vi "PH_Sixpack.ProcCases.vi"(0 "i ref in":refnum<vi>, 1 "selector":string, 2 "Data":T1, 3 "call cluster":T2={"Object"="", "Selector"="", "CallType"=enum."synchronous", "Async Object"="", "Async Selector"="", "Data Descriptor"="", "Data"=[], "Error #"=0, "Expire"=0}, 5 "error in":errorcluster) -> (14 "i ref out":refnum<vi>, 17 "answer cluster":T2={"Object"="", "Selector"="", "CallType"=enum."synchronous", "Async Object"="", "Async Selector"="", "Data Descriptor"="", "Data"=[], "Error #"=0, "Expire"=0}, 19 "error out":errorcluster)   [LabVIEW 2014, in "PH_Sixpack.lvlib"]
doc: "This method is called by a process from within the default case in the event loop. The methods of a class that are linked to events will be called from THIS method. Add your code here."
uses:
  PH_Sixpack.lvlib
  CSCore/CSSystem/CoreDefs/CoreDefs.call_type.ctl
  CSCore/BaseProcess/BaseProcess.descriptor string definition.ctl
  CSCore/CSSystem/CoreDefs/CoreDefs.rawDataType.ctl
  PH_Sixpack.Status.ctl
  PH_PSDBWriter/PH_PSDBWriter.Thread Commands.ctl
  instr.lib/SixPack/PackDLL/Current Control.ctl
  instr.lib/SixPack/PackDLL/Current.ctl
  instr.lib/SixPack/PackDLL/VStartVmin.ctl
  instr.lib/SixPack/PackDLL/VmaxAmax.ctl
  instr.lib/SixPack/PackDLL/MotorParameter_P5.ctl
  instr.lib/SixPack/PackDLL/MotorParameter_P6.ctl
  instr.lib/SixPack/PackDLL/Motor Parameter.ctl
  instr.lib/SixPack/PackDLL/Ref Search Parameter.ctl
  instr.lib/SixPack/PackDLL/Stopswitch Limits.ctl
  CSCore/CSSystem/CoreLib/CoreLib.string 2 byte array.vi
  CSCore/CSSystem/CoreLib/CoreLib.byte array 2 int.vi
  CSCore/CSSystem/CoreLib/CoreLib.byte array 2 double.vi
  CSCore/CSSystem/CoreLib/CoreLib.lvlib
  CSCore/BaseProcess/BaseProcess.lvlib
  CSCore/CAEObj/CAEObj.lvlib
  PH_PSDBWriter/PH_PSDBWriter.lvlib
  PH_Stepmotor_BaseClass/PH_Stepmotor_BaseClass.lvlib
  instr.lib/SixPack/Sixpack - Driver.lvlib
  CSCore/CSSystem/CSSystemLib/CSSystemLib.lvlib
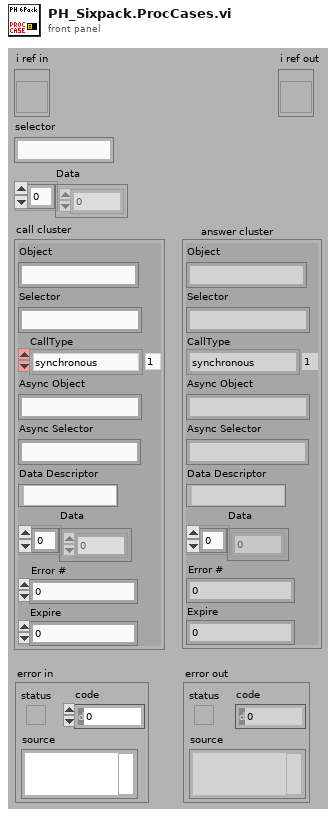
[diagram p1: front panel]
types:
  T1 = typedef "CoreDefs.rawDataType.ctl" = i8[]
  T2 = typedef "CoreDefs.call_type.ctl" = cluster{"Object":string, "Selector":string, "CallType":enum16{"simple", "synchronous", "asynchronous"}, "Async Object":string, "Async Selector":string, "Data Descriptor":T3, "Data":T1, "Error #":i32, "Expire":u32}
  T3 = typedef "BaseProcess.lvlib/BaseProcess.descriptor string definition.ctl" = string
  T4 = typedef "PH_Sixpack.lvlib/PH_Sixpack.Status.ctl" = enum32{"None", "Init", "Configure", "configured", "Close", "closed"}
  T5 = typedef "Sixpack - Driver.lvlib/Current Control.ctl" = cluster{"PowerDownDelay (500)":u16, "PowerDown (0%)":T6, "Standing (50%)":T6, "Running (75%)":T6, "Accelerating (100%)":T6}
  T6 = typedef "Sixpack - Driver.lvlib/Current.ctl" = enum8{"100%", "75%", "50%", "38%", "25%", "19%", "13%", "9%", "0%"}
  T7 = typedef "Sixpack - Driver.lvlib/VStartVmin.ctl" = cluster{"VStart(5)":u16, "Vmin(4)":u16, "Div i (2)":enum8{"0", "1", "2", "3"}}
  T8 = typedef "Sixpack - Driver.lvlib/VmaxAmax.ctl" = cluster{"VMax(511)":u16, "AMax(128)":u16}
  T9 = typedef "Sixpack - Driver.lvlib/Motor Parameter.ctl" = cluster{"Poslimit (6400)":u32, "P5 Bits":T10, "P6 Bits":T11}
  T10 = typedef "Sixpack - Driver.lvlib/MotorParameter_P5.ctl" = cluster{"MT_PI":bool, "MT_ROTARY":bool, "MT_AUTONULLCMD":bool, "MT_TESTNULL":bool, "MT_NULLLEFT":bool, "MT_NULLCENTRE":bool, "MT_STOPNULL":bool, "MT_FILTERSWITCH":bool}
  T11 = typedef "Sixpack - Driver.lvlib/MotorParameter_P6.ctl" = cluster{"MT_OPTIMIZEWAY":bool, "MT_FASTREF":bool, "MT_MECHREF":bool, "MT_DELAYTESTNULL":bool, "MT_STOPSOFT":bool, "MT_STOPNOREF":bool, "MT_NULLPOSITIVE":bool, "MUT_STOPFULSTEPS":bool}
  T12 = typedef "Sixpack - Driver.lvlib/Ref Search Parameter.ctl" = cluster{"VRefMax(100)":u16, "DebouncingTime (22ms)":u8}
  T13 = typedef "Sixpack - Driver.lvlib/Stopswitch Limits.ctl" = cluster{"MinLeft(0)":u16, "MaxRight(1023)":u16}
  T14 = typedef "PH_PSDBWriter.lvlib/PH_PSDBWriter.PHELIX-Subsystems.ctl" = i32
  T15 = typedef "PH_PSDBWriter.lvlib/PH_PSDBWriter.Thread Commands.ctl" = u16
  T16 = typedef "PH_Stepmotor_BaseClass.lvlib/PH_Stepmotor_BaseClass.i attribute.ctl" = cluster{"Device Error":errorcluster, "Axes PSDB Thread":cluster{"Ref":refnum<vi>, "Q-Ref":refnum<queue>, "Data Status":T17}, "Axes":T18[], "Axes PSDB Infos":cluster{"GUI Name":string, "PSDB Instance ID":i32, "PSDB Status Service ID":i32, "Axis":i32, "Class":string}[], "GUI Refs":T23}
  T17 = typedef "PH_PSDBWriter.lvlib/PH_PSDBWriter.Data Status.ctl" = i16
  T18 = typedef "PH_Stepmotor_BaseClass.lvlib/PH_Stepmotor_BaseClass.Axis Attributes.ctl" = cluster{"Settings":T19, "Endswitch?":bool, "DIM Service IDs":T21, "Activity":T22, "Configured?":bool, "Position":cluster{"Current":i32, "Target":i32}, "Position to set":cluster{"New?":bool, "Wanted":i32}, "Stop?":bool, "Reset?":bool, "Move?":bool, "Nothing connected?":bool}
  T19 = typedef "PH_Stepmotor_BaseClass.lvlib/PH_Stepmotor_BaseClass.Axis Settings.ctl" = cluster{"Sign change":bool, "Width":dbl, "Calibration":dbl, "Unit":string, "Motor Type":T20, "Unit Width":string, "Unit CF":string}
  T20 = typedef "PH_Stepmotor_BaseClass.lvlib/PH_Stepmotor_BaseClass.Motor Type.ctl" = enum16{"Unspecific", "OWIS 49.120.2633", "OWIS 49.060.1033", "OWIS 43.040.2558", "Diamond Motion 2200 series", "OWIS 49.120.266B.MV6", "Calorimeter", "Linear Stage 1", "MICOS VT-80", "MICOS VT-80 S", "Standa Rotstage nt0.95A", "PUF RA 320.200", "PUF RA 800.200", "PUF RA 800.400", "PUF RA 400.50", "1324.nn.800.50", "1324.n9c.800.50", "1324.nn.320.200", "1324.nn.400.200", "1324.nn.800.200", "1324.nn.400.50", "1324.8c9c.800.50", "1324.8c9c.400.200"}
  T21 = typedef "PH_Stepmotor_BaseClass.lvlib/PH_Stepmotor_BaseClass.Axis DIM Service IDs.ctl" = cluster{"Settings":i32, "Information":i32}
  T22 = typedef "PH_Stepmotor_BaseClass.lvlib/PH_Stepmotor_BaseClass.Axis Activity.ctl" = enum16{"No Information", "stopped", "running", "Failure", "Alarm", "stopped at backward ES", "stopped at foreward ES"}
  T23 = typedef "PH_Stepmotor_BaseClass.lvlib/PH_Stepmotor_BaseClass.GUI Refs.ctl" = cluster{"Axes Configuration":refnum<vi>, "Device Error":refnum<vi>, "Axes PSDB Infos":refnum<vi>}
  T24 = cluster{"Boolean array[0]":bool, "Boolean array[1]":bool, "Boolean array[2]":bool, "Boolean array[3]":bool, "Boolean array[4]":bool, "Boolean array[5]":bool, "Boolean array[6]":bool, "Boolean array[7]":bool}
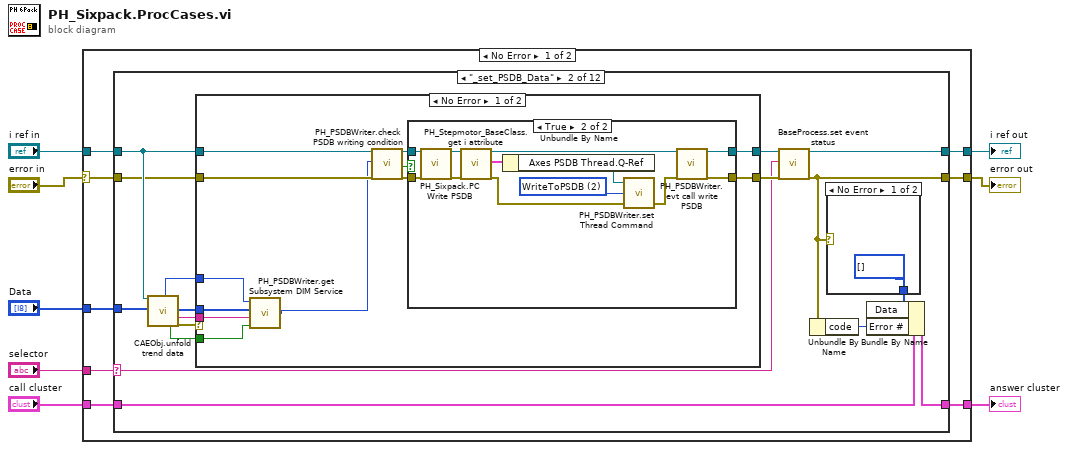
[diagram p0: block diagram]
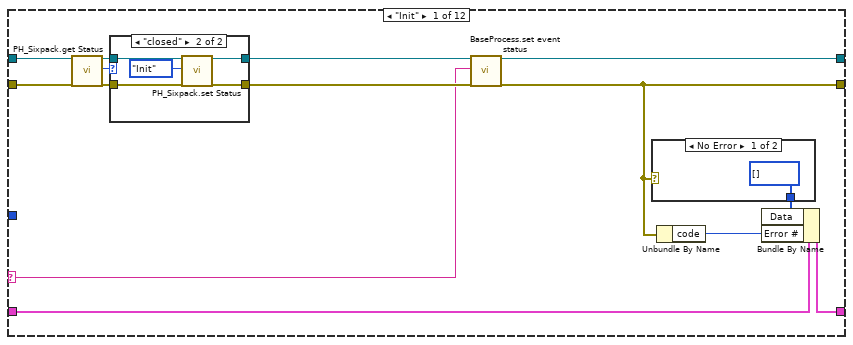
[diagram p2: hidden frame]
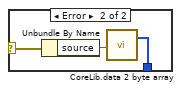
[diagram p4: hidden frame]
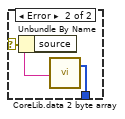
[diagram p7: hidden frame]
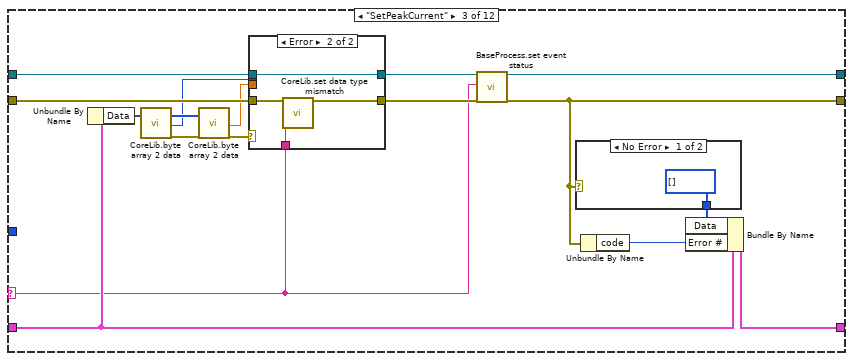
[diagram p8: hidden frame]
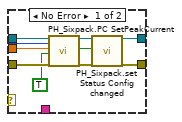
[diagram p9: hidden frame]
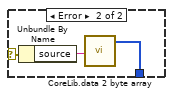
[diagram p10: hidden frame]
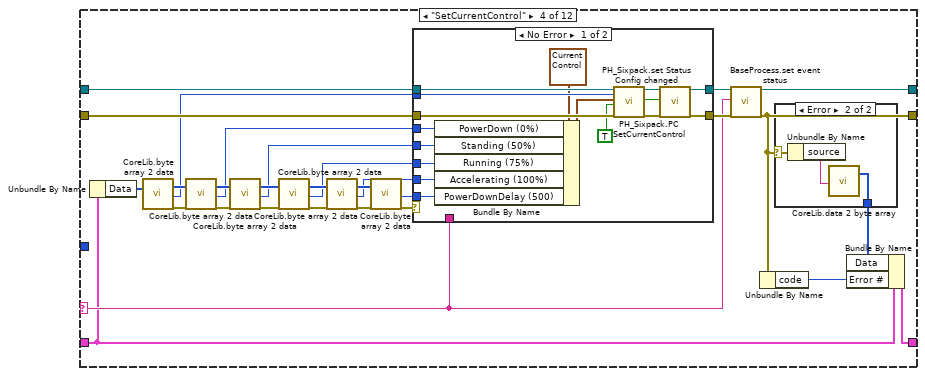
[diagram p11: hidden frame]
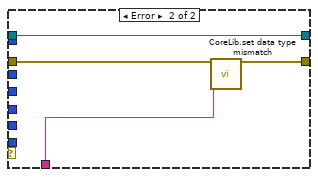
[diagram p12: hidden frame]
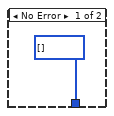
[diagram p13: hidden frame]
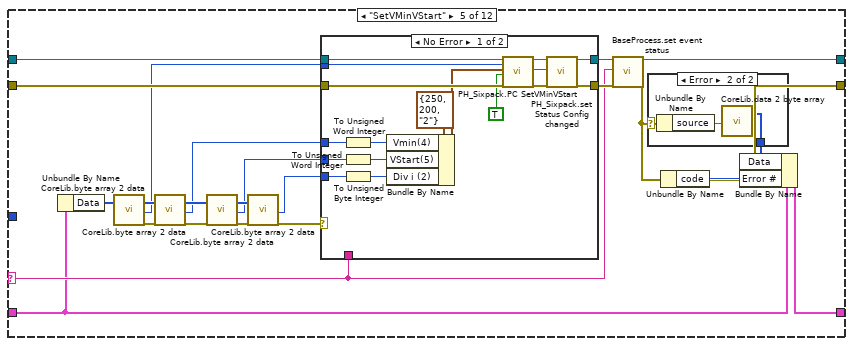
[diagram p14: hidden frame]
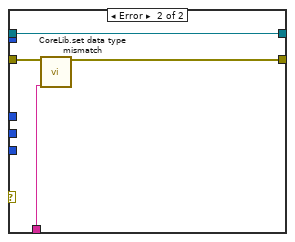
[diagram p15: hidden frame]
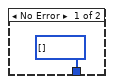
[diagram p16: hidden frame]
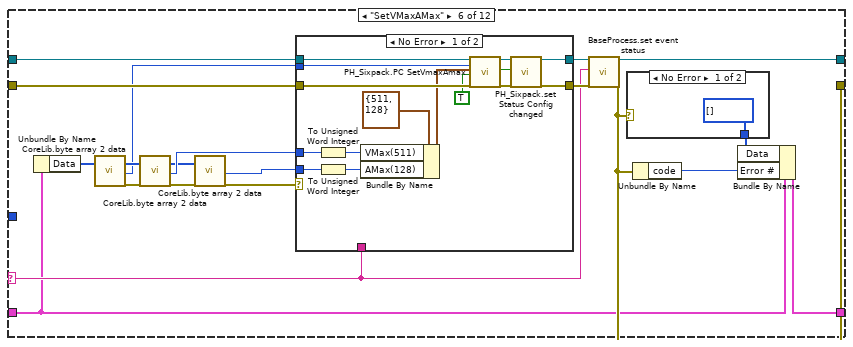
[diagram p17: hidden frame]
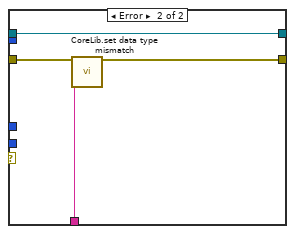
[diagram p18: hidden frame]
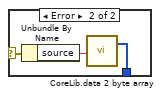
[diagram p19: hidden frame]
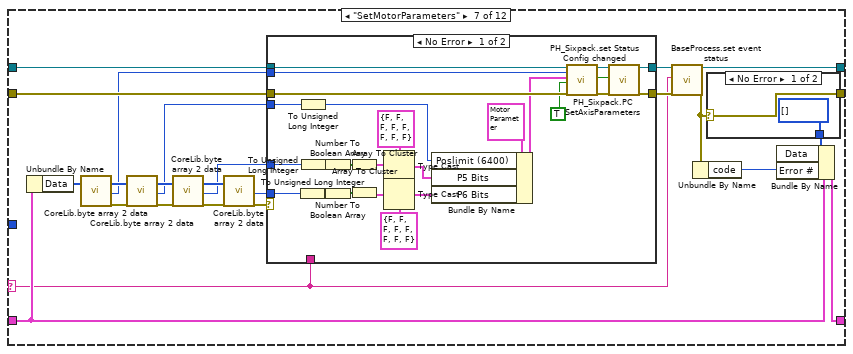
[diagram p20: hidden frame]
diagram:
  n1 = case shown="No Error" "error in" {
    selector: "error in" -> [w11 w500]
    tunnel: [w16 w499] -> w8
    tunnel: [w9 w500] -> w7
    tunnel: "call cluster" -> [w15 w499]
    tunnel: "selector" -> [w14 _]
    tunnel: [w10 w501] -> w4
    tunnel: "i ref in" -> [w13 w501]
    tunnel: "Data" -> [w12 _]
    frame No Error {
      n2 = case shown="\"_set_PSDB_Data\"" w14 {
        selector: w14 -> [w22 w43 w99 w149 w194 w239 w270 w337 w382 w419 w458 w474]
        tunnel: [w25 w56 w104 w151 w198 w242 w289 w342 w385 w422 w459 w484] -> w10
        tunnel: w15 -> [w30 w44 w100 w148 w193 w238 w286 w341 w381 w418 w462 w486]
        tunnel: [w29 w58 w102 w147 w195 w246 w287 w340 w369 w413 w461 w489] -> w16
        tunnel: w11 -> [w27 w47 w103 w150 w197 w244 w288 w339 w384 w421 w455 w490]
        tunnel: [w23 w55 w101 w146 w196 w240 w273 w338 w383 w420 w456 w482] -> w9
        tunnel: w13 -> [w19 w48 w98 w145 w192 w237 w285 w336 w380 w417 w452 w488]
        tunnel: w12 -> [_ w42 _ _ _ _ _ _ _ _ _ w487]
        frame "Init" {
          n3 = call "PH_Sixpack.get Status.vi"("VI in"=w19, "error in (no error)"=w27) -> ("VI out"=w18:refnum<vi>, "Status"=w17:T4, "Device Error"=w20:errorcluster)  [unwired: 14 in, 1 out]
          n4 = case shown="\"closed\"" w17 {
            tunnel: [w32 w37] -> w26
            tunnel: [w31 w36] -> w24
            tunnel: w20 -> [w31 w34]
            tunnel: w18 -> [w32 w33]
            frame "None", Default {
            }
            frame "closed" {
              n5 = call "PH_Sixpack.set Status.vi"("VI in"=w33, "Status"=PH_Sixpack.Status."Init", "error in (no error)"=w34) -> ("VI out"=w37:refnum<vi>, "error out"=w36:errorcluster)  [unwired: 15 in]
            }
          }
          n6 = call "BaseProcess.set event status.vi"("i ref in"=w26, "EventStatus"=w22, "error in (no error)"=w24) -> ("i ref out"=w25:refnum<vi>, "error out"=w23:errorcluster)  [unwired: 14 in, 1 out]
          n7 = case shown="No Error" w23 {
            selector: w23 -> [_ w41]
            tunnel: [T1 [] ("byteArray out") w39] -> w21
            frame No Error {
            }
            frame Error {
              n8 = Unbundle By Name(w41) -> ("source"=w40:string)
              n9 = call-poly "CoreLib.data 2 byte array.vi"("string"=w40) -> ("byteArray out"=w39:T1)  [unwired: 18 in]
            }
          }
          n10 = Unbundle By Name(w23) -> ("code"=w28:i32)
          n11 = Bundle By Name(cluster=w30, "Data"=w21, "Error #"=w28) -> (w29:T2)
        }
        frame "_set_PSDB_Data" {
          n12 = call "CAEObj.unfold trend data.vi"("i ref in"=w48, "raw trend data"=w42) -> ("quality"=w49:i32, "no link"=w52:bool, "data"=w50:i8[], "typeDescriptor"=w51:string, "error out"=w53:errorcluster)  [unwired: 9 in, 4 out]
          n13 = case shown="No Error" w53 {
            tunnel: w47 -> [w70 w86]
            tunnel: [w69 w85] -> w46
            tunnel: [w68 w86] -> w45
            tunnel: w48 -> [w66 w85]
            tunnel: w52 -> [w60 _]
            tunnel: w51 -> [w61 _]
            tunnel: w50 -> [w63 _]
            tunnel: w49 -> [w62 _]
            frame No Error {
              n14 = call "PH_PSDBWriter.get Subsystem DIM Service.vi"("no link"=w60, "typeDescriptor"=w61, "data"=w63, "quality"=w62) -> ("PHELIX Subsystems"=w59:T14)
              n15 = call "PH_PSDBWriter.check PSDB writing condition.vi"("i ref in"=w66, "wanted Subsystem"=w59, "error IO"=w70) -> ("i ref out"=w65:refnum<vi>, "write PSDB?"=w64:bool, "error out"=w67:errorcluster)  [unwired: 14 in]
              n16 = case shown="True" w64 {
                tunnel: w67 -> [w71 w84]
                tunnel: [w72 w75] -> w69
                tunnel: [w71 w73] -> w68
                tunnel: w65 -> [w72 w83]
                frame False {
                }
                frame True {
                  w79 = T15 2 items=["None", "GetInstanceID", "WriteToPSDB"] ("PSDB Thread Command")
                  n17 = call "PH_Sixpack.PC Write PSDB.vi"("i ref in"=w83, "error IO"=w84) -> ("i ref out"=w77:refnum<vi>, "error out"=w78:errorcluster)  [unwired: 16 in]
                  n18 = call "PH_Stepmotor_BaseClass.get i attribute.vi"("i ref in"=w77, "error in (no error)"=w78) -> ("i ref out"=w76:refnum<vi>, "i attribute"=w81:T16, "error out"=w82:errorcluster)  [unwired: 15 in]
                  n19 = Unbundle By Name(w81) -> ("Axes PSDB Thread.Q-Ref"=w80:refnum<queue>)
                  n20 = call "PH_PSDBWriter.set Thread Command.vi"("error in (no error)"=w82, "PSDB Thread Command"=w79, "Queue in"=w80) -> ("error out"=w74:errorcluster)  [unwired: 2 in]
                  n21 = call "PH_PSDBWriter.evt call write PSDB.vi"("i ref in"=w76, "error in (no error)"=w74) -> ("i ref out"=w75:refnum<vi>, "error out"=w73:errorcluster)  [unwired: 16 in]
                }
              }
            }
            frame Error {
            }
          }
          n22 = call "BaseProcess.set event status.vi"("i ref in"=w46, "EventStatus"=w43, "error in (no error)"=w45) -> ("i ref out"=w56:refnum<vi>, "error out"=w55:errorcluster)  [unwired: 14 in, 1 out]
          n23 = Unbundle By Name(w55) -> ("code"=w57:i32)
          n24 = case shown="No Error" w55 {
            selector: w55 -> [_ w90]
            tunnel: [T1 [] ("byteArray out") w88] -> w54
            frame No Error {
            }
            frame Error {
              n25 = Unbundle By Name(w90) -> ("source"=w89:string)
              n26 = call-poly "CoreLib.data 2 byte array.vi"("string"=w89) -> ("byteArray out"=w88:T1)  [unwired: 18 in]
            }
          }
          n27 = Bundle By Name(cluster=w44, "Data"=w54, "Error #"=w57) -> (w58:T2)
        }
        frame "SetPeakCurrent" {
          n28 = Unbundle By Name(w100) -> ("Data"=w92:T1)
          n29 = call-poly "CoreLib.byte array 2 data.vi"("byteArray"=w92) -> ("byteArray out"=w96:T1, "i32"=w95:i32, "error out"=w97:errorcluster)  [unwired: 16 in]
          n30 = call-poly "CoreLib.byte array 2 data.vi"("byteArray"=w96, "error in (no error)"=w97) -> ("d64"=w94:dbl, "error out"=w93:errorcluster)  [unwired: 15 in, 1 out]
          n31 = case shown="Error" w93 {
            tunnel: [w110 w118] -> w106
            tunnel: [w112 w120] -> w105
            tunnel: w103 -> [w116 w121]
            tunnel: w95 -> [w115 _]
            tunnel: w94 -> [w114 _]
            tunnel: w99 -> [_ w119]
            tunnel: w98 -> [w113 w118]
            frame No Error {
              n32 = call "PH_Sixpack.PC SetPeakCurrent.vi"("i ref in"=w113, "Axis"=w115, "Imax (50%)"=w114, "To set?"=TRUE, "error in"=w116) -> ("i ref out"=w111:refnum<vi>, "ok?"=w108:bool, "error out"=w117:errorcluster)  [unwired: 12 in]
              n33 = call "PH_Sixpack.set Status Config changed.vi"("VI in"=w111, "Config changed?"=w108, "error in"=w117) -> ("VI out"=w110:refnum<vi>, "error out"=w112:errorcluster)  [unwired: 15 in]
            }
            frame Error {
              n34 = call "CoreLib.set data type mismatch.vi"("error in (no error)"=w121, "error source"=w119) -> ("error out"=w120:errorcluster)  [unwired: 17 in]
            }
          }
          n35 = call "BaseProcess.set event status.vi"("i ref in"=w106, "EventStatus"=w99, "error in (no error)"=w105) -> ("i ref out"=w104:refnum<vi>, "error out"=w101:errorcluster)  [unwired: 14 in, 1 out]
          n36 = case shown="No Error" w101 {
            selector: w101 -> [_ w125]
            tunnel: [T1 [] ("byteArray out") w123] -> w91
            frame No Error {
            }
            frame Error {
              n37 = Unbundle By Name(w125) -> ("source"=w124:string)
              n38 = call-poly "CoreLib.data 2 byte array.vi"("string"=w124) -> ("byteArray out"=w123:T1)  [unwired: 18 in]
            }
          }
          n39 = Unbundle By Name(w101) -> ("code"=w107:i32)
          n40 = Bundle By Name(cluster=w100, "Data"=w91, "Error #"=w107) -> (w102:T2)
        }
        frame "SetCurrentControl" {
          n41 = Unbundle By Name(w148) -> ("Data"=w127:T1)
          n42 = call-poly "CoreLib.byte array 2 data.vi"("byteArray"=w127) -> ("byteArray out"=w140:T1, "i32"=w134:i32, "error out"=w138:errorcluster)  [unwired: 16 in]
          n43 = call-poly "CoreLib.byte array 2 data.vi"("byteArray"=w140, "error in (no error)"=w138) -> ("byteArray out"=w139:T1, "i32"=w133:i32, "error out"=w137:errorcluster)  [unwired: 15 in]
          n44 = call-poly "CoreLib.byte array 2 data.vi"("byteArray"=w139, "error in (no error)"=w137) -> ("byteArray out"=w141:T1, "i32"=w132:i32, "error out"=w136:errorcluster)  [unwired: 15 in]
          n45 = call-poly "CoreLib.byte array 2 data.vi"("byteArray"=w141, "error in (no error)"=w136) -> ("byteArray out"=w142:T1, "i32"=w131:i32, "error out"=w135:errorcluster)  [unwired: 15 in]
          n46 = call-poly "CoreLib.byte array 2 data.vi"("byteArray"=w142, "error in (no error)"=w135) -> ("byteArray out"=w144:T1, "i32"=w130:i32, "error out"=w143:errorcluster)  [unwired: 15 in]
          n47 = call-poly "CoreLib.byte array 2 data.vi"("byteArray"=w144, "error in (no error)"=w143) -> ("i32"=w129:i32, "error out"=w128:errorcluster)  [unwired: 15 in, 1 out]
          n48 = case shown="No Error" w128 {
            tunnel: [w166 w171] -> w153
            tunnel: [w164 w173] -> w152
            tunnel: w150 -> [w170 w174]
            tunnel: w134 -> [w169 _]
            tunnel: w133 -> [w157 _]
            tunnel: w149 -> [_ w172]
            tunnel: w132 -> [w158 _]
            tunnel: w131 -> [w159 _]
            tunnel: w145 -> [w168 w171]
            tunnel: w130 -> [w160 _]
            tunnel: w129 -> [w161 _]
            frame No Error {
              n49 = Bundle By Name(cluster=T5 {"PowerDownDelay (500)"=500, "PowerDown (0%)"=enum."0%", "Standing (50%)"=enum."50%", "Running (75%)"=enum."75%", "Accelerating (100%)"=enum."100%"} ("Wanted I Control"), "PowerDown (0%)"=w157, "Standing (50%)"=w158, "Running (75%)"=w159, "Accelerating (100%)"=w160, "PowerDownDelay (500)"=w161) -> (w162:T5)
              n50 = call "PH_Sixpack.PC SetCurrentControl.vi"("i ref in"=w168, "axis"=w169, "Wanted I Control"=w162, "To set?"=TRUE, "error in"=w170) -> ("i ref out"=w167:refnum<vi>, "ok?"=w155:bool, "error out"=w165:errorcluster)  [unwired: 12 in]
              n51 = call "PH_Sixpack.set Status Config changed.vi"("VI in"=w167, "Config changed?"=w155, "error in"=w165) -> ("VI out"=w166:refnum<vi>, "error out"=w164:errorcluster)  [unwired: 15 in]
            }
            frame Error {
              n52 = call "CoreLib.set data type mismatch.vi"("error in (no error)"=w174, "error source"=w172) -> ("error out"=w173:errorcluster)  [unwired: 17 in]
            }
          }
          n53 = call "BaseProcess.set event status.vi"("i ref in"=w153, "EventStatus"=w149, "error in (no error)"=w152) -> ("i ref out"=w151:refnum<vi>, "error out"=w146:errorcluster)  [unwired: 14 in, 1 out]
          n54 = Unbundle By Name(w146) -> ("code"=w154:i32)
          n55 = case shown="Error" w146 {
            selector: w146 -> [_ w178]
            tunnel: [T1 [] ("byteArray out") w176] -> w126
            frame No Error {
            }
            frame Error {
              n56 = Unbundle By Name(w178) -> ("source"=w177:string)
              n57 = call-poly "CoreLib.data 2 byte array.vi"("string"=w177) -> ("byteArray out"=w176:T1)  [unwired: 18 in]
            }
          }
          n58 = Bundle By Name(cluster=w148, "Data"=w126, "Error #"=w154) -> (w147:T2)
        }
        frame "SetVMinVStart" {
          n59 = Unbundle By Name(w193) -> ("Data"=w180:T1)
          n60 = call-poly "CoreLib.byte array 2 data.vi"("byteArray"=w180) -> ("byteArray out"=w190:T1, "i32"=w182:i32, "error out"=w189:errorcluster)  [unwired: 16 in]
          n61 = call-poly "CoreLib.byte array 2 data.vi"("byteArray"=w190, "error in (no error)"=w189) -> ("byteArray out"=w186:T1, "i32"=w183:i32, "error out"=w185:errorcluster)  [unwired: 15 in]
          n62 = call-poly "CoreLib.byte array 2 data.vi"("byteArray"=w186, "error in (no error)"=w185) -> ("byteArray out"=w187:T1, "i32"=w184:i32, "error out"=w188:errorcluster)  [unwired: 15 in]
          n63 = call-poly "CoreLib.byte array 2 data.vi"("byteArray"=w187, "error in (no error)"=w188) -> ("i32"=w179:i32, "error out"=w181:errorcluster)  [unwired: 15 in, 1 out]
          n64 = case shown="No Error" w181 {
            tunnel: w197 -> [w216 w219]
            tunnel: [w214 w221] -> w200
            tunnel: [w212 w222] -> w199
            tunnel: w182 -> [w217 _]
            tunnel: w183 -> [w209 _]
            tunnel: w194 -> [_ w220]
            tunnel: w184 -> [w208 _]
            tunnel: w179 -> [w206 _]
            tunnel: w192 -> [w218 w221]
            frame No Error {
              n65 = To Unsigned Word Integer(number=w209) -> (unsigned 16bit integer=w204:u16)
              n66 = To Unsigned Word Integer(number=w208) -> (unsigned 16bit integer=w205:u16)
              n67 = To Unsigned Byte Integer(number=w206) -> (unsigned 8bit integer=w207:u8)
              n68 = Bundle By Name(cluster=T7 {"VStart(5)"=250, "Vmin(4)"=200, "Div i (2)"=enum."2"} ("VStartVminDivi"), "Vmin(4)"=w204, "VStart(5)"=w205, "Div i (2)"=w207) -> (w210:T7)
              n69 = call "PH_Sixpack.PC SetVMinVStart.vi"("i ref in"=w218, "axis"=w217, "VStartVminDivi"=w210, "To Set?"=TRUE, "error in (no error)"=w216) -> ("i ref out"=w215:refnum<vi>, "ok?"=w202:bool, "error out"=w213:errorcluster)  [unwired: 12 in]
              n70 = call "PH_Sixpack.set Status Config changed.vi"("VI in"=w215, "Config changed?"=w202, "error in"=w213) -> ("VI out"=w214:refnum<vi>, "error out"=w212:errorcluster)  [unwired: 15 in]
            }
            frame Error {
              n71 = call "CoreLib.set data type mismatch.vi"("error in (no error)"=w219, "error source"=w220) -> ("error out"=w222:errorcluster)  [unwired: 17 in]
            }
          }
          n72 = call "BaseProcess.set event status.vi"("i ref in"=w200, "EventStatus"=w194, "error in (no error)"=w199) -> ("i ref out"=w198:refnum<vi>, "error out"=w196:errorcluster)  [unwired: 14 in, 1 out]
          n73 = case shown="Error" w196 {
            selector: w196 -> [_ w226]
            tunnel: [T1 [] ("byteArray out") w224] -> w191
            frame No Error {
            }
            frame Error {
              n74 = Unbundle By Name(w226) -> ("source"=w225:string)
              n75 = call-poly "CoreLib.data 2 byte array.vi"("string"=w225) -> ("byteArray out"=w224:T1)  [unwired: 18 in]
            }
          }
          n76 = Unbundle By Name(w196) -> ("code"=w201:i32)
          n77 = Bundle By Name(cluster=w193, "Data"=w191, "Error #"=w201) -> (w195:T2)
        }
        frame "SetVMaxAMax" {
          n78 = Unbundle By Name(w238) -> ("Data"=w232:T1)
          n79 = call-poly "CoreLib.byte array 2 data.vi"("byteArray"=w232) -> ("byteArray out"=w236:T1, "i32"=w234:i32, "error out"=w235:errorcluster)  [unwired: 16 in]
          n80 = call-poly "CoreLib.byte array 2 data.vi"("byteArray"=w236, "error in (no error)"=w235) -> ("byteArray out"=w228:T1, "i32"=w233:i32, "error out"=w230:errorcluster)  [unwired: 15 in]
          n81 = call-poly "CoreLib.byte array 2 data.vi"("byteArray"=w228, "error in (no error)"=w230) -> ("i32"=w227:i32, "error out"=w229:errorcluster)  [unwired: 15 in, 1 out]
          n82 = case shown="No Error" w229 {
            tunnel: w244 -> [w261 w264]
            tunnel: [w256 w262] -> w243
            tunnel: [w255 w265] -> w241
            tunnel: w234 -> [w260 _]
            tunnel: w233 -> [w250 _]
            tunnel: w239 -> [_ w263]
            tunnel: w237 -> [w259 w262]
            tunnel: w227 -> [w252 _]
            frame No Error {
              n83 = To Unsigned Word Integer(number=w250) -> (unsigned 16bit integer=w249:u16)
              n84 = To Unsigned Word Integer(number=w252) -> (unsigned 16bit integer=w251:u16)
              n85 = Bundle By Name(cluster=T8 {"VMax(511)"=511, "AMax(128)"=128} ("V Max"), "VMax(511)"=w249, "AMax(128)"=w251) -> (w253:T8)
              n86 = call "PH_Sixpack.PC SetVmaxAmax.vi"("i ref in"=w259, "axis"=w260, "V max A max"=w253, "To Set?"=TRUE, "error in"=w261) -> ("i ref out"=w257:refnum<vi>, "ok?"=w247:bool, "error out"=w258:errorcluster)  [unwired: 12 in]
              n87 = call "PH_Sixpack.set Status Config changed.vi"("VI in"=w257, "Config changed?"=w247, "error in"=w258) -> ("VI out"=w256:refnum<vi>, "error out"=w255:errorcluster)  [unwired: 15 in]
            }
            frame Error {
              n88 = call "CoreLib.set data type mismatch.vi"("error in (no error)"=w264, "error source"=w263) -> ("error out"=w265:errorcluster)  [unwired: 17 in]
            }
          }
          n89 = call "BaseProcess.set event status.vi"("i ref in"=w243, "EventStatus"=w239, "error in (no error)"=w241) -> ("i ref out"=w242:refnum<vi>, "error out"=w240:errorcluster)  [unwired: 14 in, 1 out]
          n90 = case shown="No Error" w240 {
            selector: w240 -> [_ w269]
            tunnel: [T1 [] ("byteArray out") w267] -> w231
            frame No Error {
            }
            frame Error {
              n91 = Unbundle By Name(w269) -> ("source"=w268:string)
              n92 = call-poly "CoreLib.data 2 byte array.vi"("string"=w268) -> ("byteArray out"=w267:T1)  [unwired: 18 in]
            }
          }
          n93 = Unbundle By Name(w240) -> ("code"=w245:i32)
          n94 = Bundle By Name(cluster=w238, "Data"=w231, "Error #"=w245) -> (w246:T2)
        }
        frame "SetMotorParameters" {
          n95 = Unbundle By Name(w286) -> ("Data"=w278:T1)
          n96 = call-poly "CoreLib.byte array 2 data.vi"("byteArray"=w278) -> ("byteArray out"=w284:T1, "i32"=w277:i32, "error out"=w279:errorcluster)  [unwired: 16 in]
          n97 = call-poly "CoreLib.byte array 2 data.vi"("byteArray"=w284, "error in (no error)"=w279) -> ("byteArray out"=w283:T1, "i32"=w272:i32, "error out"=w280:errorcluster)  [unwired: 15 in]
          n98 = call-poly "CoreLib.byte array 2 data.vi"("byteArray"=w283, "error in (no error)"=w280) -> ("byteArray out"=w282:T1, "i32"=w276:i32, "error out"=w281:errorcluster)  [unwired: 15 in]
          n99 = call-poly "CoreLib.byte array 2 data.vi"("byteArray"=w282, "error in (no error)"=w281) -> ("i32"=w275:i32, "error out"=w271:errorcluster)  [unwired: 15 in, 1 out]
          n100 = case shown="No Error" w271 {
            tunnel: [w297 w321] -> w291
            tunnel: [w295 w319] -> w290
            tunnel: w288 -> [w317 w320]
            tunnel: w285 -> [w316 w321]
            tunnel: w277 -> [w307 _]
            tunnel: w276 -> [w306 _]
            tunnel: w275 -> [w305 _]
            tunnel: w272 -> [w300 _]
            tunnel: w270 -> [_ w318]
            frame No Error {
              n101 = To Unsigned Long Integer(number=w305) -> (unsigned 32bit integer=w312:u32)
              n102 = To Unsigned Long Integer(number=w300) -> (unsigned 32bit integer=w299:u32)
              n103 = To Unsigned Long Integer(number=w306) -> (unsigned 32bit integer=w313:u32)
              n104 = Number To Boolean Array(number=w313) -> (Boolean array=w315:bool[])
              n105 = Number To Boolean Array(number=w312) -> (Boolean array=w314:bool[])
              n106 = Array To Cluster(array=w315) -> (cluster=w309:T24)
              n107 = Array To Cluster(array=w314) -> (cluster=w311:T24)
              n108 = Type Cast(type=T10 {"MT_PI"=FALSE, "MT_ROTARY"=FALSE, "MT_AUTONULLCMD"=FALSE, "MT_TESTNULL"=FALSE, "MT_NULLLEFT"=FALSE, "MT_NULLCENTRE"=FALSE, "MT_STOPNULL"=FALSE, "MT_FILTERSWITCH"=FALSE} ("P5 Bits"), x=w309) -> (*(type *) &x=w301:T10)
              n109 = Type Cast(type=T11 {"MT_OPTIMIZEWAY"=FALSE, "MT_FASTREF"=FALSE, "MT_MECHREF"=FALSE, "MT_DELAYTESTNULL"=FALSE, "MT_STOPSOFT"=FALSE, "MT_STOPNOREF"=FALSE, "MT_NULLPOSITIVE"=FALSE, "MUT_STOPFULSTEPS"=FALSE} ("P6 Bits"), x=w311) -> (*(type *) &x=w302:T11)
              n110 = Bundle By Name(cluster=T9 {"Poslimit (6400)"=6400, "P5 Bits"={"MT_PI"=FALSE, "MT_ROTARY"=FALSE, "MT_AUTONULLCMD"=FALSE, "MT_TESTNULL"=FALSE, "MT_NULLLEFT"=FALSE, "MT_NULLCENTRE"=FALSE, "MT_STOPNULL"=FALSE, "MT_FILTERSWITCH"=FALSE}, "P6 Bits"={"MT_OPTIMIZEWAY"=FALSE, "MT_FASTREF"=FALSE, "MT_MECHREF"=FALSE, "MT_DELAYTESTNULL"=FALSE, "MT_STOPSOFT"=FALSE, "MT_STOPNOREF"=FALSE, "MT_NULLPOSITIVE"=FALSE, "MUT_STOPFULSTEPS"=FALSE}} ("Axis Parameter"), "Poslimit (6400)"=w299, "P5 Bits"=w301, "P6 Bits"=w302) -> (w303:T9)
              n111 = call "PH_Sixpack.PC SetAxisParameters.vi"("i ref in"=w316, "axis"=w307, "Axis Parameter"=w303, "Set?"=TRUE, "error in (no error)"=w317) -> ("i ref out"=w298:refnum<vi>, "ok?"=w293:bool, "error out"=w296:errorcluster)  [unwired: 12 in]
              n112 = call "PH_Sixpack.set Status Config changed.vi"("VI in"=w298, "Config changed?"=w293, "error in"=w296) -> ("VI out"=w297:refnum<vi>, "error out"=w295:errorcluster)  [unwired: 15 in]
            }
            frame Error {
              n113 = call "CoreLib.set data type mismatch.vi"("error in (no error)"=w320, "error source"=w318) -> ("error out"=w319:errorcluster)  [unwired: 17 in]
            }
          }
          n114 = call "BaseProcess.set event status.vi"("i ref in"=w291, "EventStatus"=w270, "error in (no error)"=w290) -> ("i ref out"=w289:refnum<vi>, "error out"=w273:errorcluster)  [unwired: 14 in, 1 out]
          n115 = Unbundle By Name(w273) -> ("code"=w292:i32)
          n116 = case shown="No Error" w273 {
            selector: w273 -> [_ w325]
            tunnel: [T1 [] ("byteArray out") w324] -> w274
            frame No Error {
            }
            frame Error {
              n117 = Unbundle By Name(w325) -> ("source"=w323:string)
              n118 = call-poly "CoreLib.data 2 byte array.vi"("string"=w323) -> ("byteArray out"=w324:T1)  [unwired: 18 in]
            }
          }
          n119 = Bundle By Name(cluster=w286, "Data"=w274, "Error #"=w292) -> (w287:T2)
        }
        frame "SetRefSearchParameters" {
          n120 = Unbundle By Name(w341) -> ("Data"=w328:T1)
          n121 = call-poly "CoreLib.byte array 2 data.vi"("byteArray"=w328) -> ("byteArray out"=w333:T1, "i32"=w331:i32, "error out"=w332:errorcluster)  [unwired: 16 in]
          n122 = call-poly "CoreLib.byte array 2 data.vi"("byteArray"=w333, "error in (no error)"=w332) -> ("byteArray out"=w334:T1, "i32"=w330:i32, "error out"=w335:errorcluster)  [unwired: 15 in]
          n123 = call-poly "CoreLib.byte array 2 data.vi"("byteArray"=w334, "error in (no error)"=w335) -> ("i32"=w329:i32, "error out"=w326:errorcluster)  [unwired: 15 in, 1 out]
          n124 = case shown="No Error" w326 {
            tunnel: w339 -> [w360 w363]
            tunnel: [w348 w361] -> w344
            tunnel: [w349 w364] -> w343
            tunnel: w331 -> [w358 _]
            tunnel: w330 -> [w354 _]
            tunnel: w337 -> [_ w362]
            tunnel: w329 -> [w355 _]
            tunnel: w336 -> [w359 w361]
            frame No Error {
              n125 = To Unsigned Word Integer(number=w354) -> (unsigned 16bit integer=w353:u16)
              n126 = To Unsigned Byte Integer(number=w355) -> (unsigned 8bit integer=w352:u8)
              n127 = Bundle By Name(cluster=T12 {"VRefMax(100)"=100, "DebouncingTime (22ms)"=34} ("Ref Search Parameter"), "VRefMax(100)"=w353, "DebouncingTime (22ms)"=w352) -> (w356:T12)
              n128 = call "PH_Sixpack.PC SetRefSearchParameters.vi"("i ref in"=w359, "axis"=w358, "Ref Search Parameter"=w356, "To set?"=TRUE, "error in"=w360) -> ("i ref out"=w350:refnum<vi>, "ok?"=w346:bool, "error out"=w351:errorcluster)  [unwired: 12 in]
              n129 = call "PH_Sixpack.set Status Config changed.vi"("VI in"=w350, "Config changed?"=w346, "error in"=w351) -> ("VI out"=w348:refnum<vi>, "error out"=w349:errorcluster)  [unwired: 15 in]
            }
            frame Error {
              n130 = call "CoreLib.set data type mismatch.vi"("error in (no error)"=w363, "error source"=w362) -> ("error out"=w364:errorcluster)  [unwired: 17 in]
            }
          }
          n131 = call "BaseProcess.set event status.vi"("i ref in"=w344, "EventStatus"=w337, "error in (no error)"=w343) -> ("i ref out"=w342:refnum<vi>, "error out"=w338:errorcluster)  [unwired: 14 in, 1 out]
          n132 = case shown="No Error" w338 {
            selector: w338 -> [_ w368]
            tunnel: [T1 [] ("byteArray out") w366] -> w327
            frame No Error {
            }
            frame Error {
              n133 = Unbundle By Name(w368) -> ("source"=w367:string)
              n134 = call-poly "CoreLib.data 2 byte array.vi"("string"=w367) -> ("byteArray out"=w366:T1)  [unwired: 18 in]
            }
          }
          n135 = Unbundle By Name(w338) -> ("code"=w345:i32)
          n136 = Bundle By Name(cluster=w341, "Data"=w327, "Error #"=w345) -> (w340:T2)
        }
        frame "SetStopSwitchLimits" {
          n137 = Unbundle By Name(w381) -> ("Data"=w373:T1)
          n138 = call-poly "CoreLib.byte array 2 data.vi"("byteArray"=w373) -> ("byteArray out"=w379:T1, "i32"=w375:i32, "error out"=w378:errorcluster)  [unwired: 16 in]
          n139 = call-poly "CoreLib.byte array 2 data.vi"("byteArray"=w379, "error in (no error)"=w378) -> ("byteArray out"=w377:T1, "i32"=w374:i32, "error out"=w376:errorcluster)  [unwired: 15 in]
          n140 = call-poly "CoreLib.byte array 2 data.vi"("byteArray"=w377, "error in (no error)"=w376) -> ("i32"=w371:i32, "error out"=w372:errorcluster)  [unwired: 15 in, 1 out]
          n141 = case shown="No Error" w372 {
            tunnel: w384 -> [w403 w406]
            tunnel: [w397 w404] -> w387
            tunnel: [w399 w407] -> w386
            tunnel: w375 -> [w402 _]
            tunnel: w374 -> [w394 _]
            tunnel: w382 -> [_ w405]
            tunnel: w380 -> [w401 w404]
            tunnel: w371 -> [w393 _]
            frame No Error {
              n142 = To Unsigned Word Integer(number=w393) -> (unsigned 16bit integer=w391:u16)
              n143 = To Unsigned Word Integer(number=w394) -> (unsigned 16bit integer=w392:u16)
              n144 = Bundle By Name(cluster=T13 {"MinLeft(0)"=150, "MaxRight(1023)"=900} ("Endswitch Limits"), "MinLeft(0)"=w392, "MaxRight(1023)"=w391) -> (w395:T13)
              n145 = call "PH_Sixpack.PC SetStopSwitchLimits.vi"("i ref in"=w401, "axis"=w402, "Stopswitch Limits"=w395, "To set?"=TRUE, "error in"=w403) -> ("i ref out"=w398:refnum<vi>, "ok?"=w389:bool, "error out"=w400:errorcluster)  [unwired: 12 in]
              n146 = call "PH_Sixpack.set Status Config changed.vi"("VI in"=w398, "Config changed?"=w389, "error in"=w400) -> ("VI out"=w397:refnum<vi>, "error out"=w399:errorcluster)  [unwired: 15 in]
            }
            frame Error {
              n147 = call "CoreLib.set data type mismatch.vi"("error in (no error)"=w406, "error source"=w405) -> ("error out"=w407:errorcluster)  [unwired: 17 in]
            }
          }
          n148 = call "BaseProcess.set event status.vi"("i ref in"=w387, "EventStatus"=w382, "error in (no error)"=w386) -> ("i ref out"=w385:refnum<vi>, "error out"=w383:errorcluster)  [unwired: 14 in, 1 out]
          n149 = case shown="No Error" w383 {
            selector: w383 -> [_ w411]
            tunnel: [T1 [] ("byteArray out") w409] -> w370
            frame No Error {
            }
            frame Error {
              n150 = Unbundle By Name(w411) -> ("source"=w410:string)
              n151 = call-poly "CoreLib.data 2 byte array.vi"("string"=w410) -> ("byteArray out"=w409:T1)  [unwired: 18 in]
            }
          }
          n152 = Unbundle By Name(w383) -> ("code"=w388:i32)
          n153 = Bundle By Name(cluster=w381, "Data"=w370, "Error #"=w388) -> (w369:T2)
        }
        frame "ReferenceSearch" {
          n154 = Unbundle By Name(w418) -> ("Data"=w415:T1)
          n155 = call-poly "CoreLib.byte array 2 data.vi"("byteArray"=w415) -> ("i32"=w416:i32, "error out"=w412:errorcluster)  [unwired: 16 in, 1 out]
          n156 = case shown="No Error" w412 {
            tunnel: w421 -> [w432 w443]
            tunnel: [w429 w441] -> w424
            tunnel: [w427 w444] -> w423
            tunnel: w416 -> [w426 _]
            tunnel: w419 -> [_ w442]
            tunnel: w417 -> [w431 w441]
            frame No Error {
              n157 = call "PH_Sixpack.PC RefSearch.vi"("i ref in"=w431, "axis"=w426, "error in (no error)"=w432) -> ("i ref out"=w430:refnum<vi>, "error out"=w428:errorcluster)  [unwired: 15 in]
              n158 = case shown="Default" w426 {
                selector: w426 -> [_ w436]
                tunnel: w430 -> [w434 w440]
                tunnel: [w434 w439] -> w429
                tunnel: w428 -> [w433 w438]
                tunnel: [w433 w437] -> w427
                frame -1 {
                }
                frame Default {
                  n159 = call "PH_Stepmotor_BaseClass.PC Move.vi"("i ref in"=w440, "axis"=w436, "Move"=TRUE, "error in (no error)"=w438) -> ("i ref out"=w439:refnum<vi>, "error out"=w437:errorcluster)  [unwired: 14 in]
                }
              }
            }
            frame Error {
              n160 = call "CoreLib.set data type mismatch.vi"("error in (no error)"=w443, "error source"=w442) -> ("error out"=w444:errorcluster)  [unwired: 17 in]
            }
          }
          n161 = call "BaseProcess.set event status.vi"("i ref in"=w424, "EventStatus"=w419, "error in (no error)"=w423) -> ("i ref out"=w422:refnum<vi>, "error out"=w420:errorcluster)  [unwired: 14 in, 1 out]
          n162 = case shown="No Error" w420 {
            selector: w420 -> [_ w448]
            tunnel: [T1 [] ("byteArray out") w446] -> w414
            frame No Error {
            }
            frame Error {
              n163 = Unbundle By Name(w448) -> ("source"=w447:string)
              n164 = call-poly "CoreLib.data 2 byte array.vi"("string"=w447) -> ("byteArray out"=w446:T1)  [unwired: 18 in]
            }
          }
          n165 = Unbundle By Name(w420) -> ("code"=w425:i32)
          n166 = Bundle By Name(cluster=w418, "Data"=w414, "Error #"=w425) -> (w413:T2)
        }
        frame "Close" {
          n167 = call "PH_Sixpack.get Status.vi"("VI in"=w452, "error in (no error)"=w455) -> ("VI out"=w451:refnum<vi>, "Status"=w450:T4, "error out"=w449:errorcluster)  [unwired: 14 in, 1 out]
          n168 = case shown="Default" w450 {
            tunnel: [w463 w469] -> w454
            tunnel: [w464 w468] -> w453
            tunnel: w449 -> [w463 w466]
            tunnel: w451 -> [w464 w465]
            frame "None", "Init", "closed" {
            }
            frame Default {
              n169 = call "PH_Sixpack.set Status.vi"("VI in"=w465, "Status"=PH_Sixpack.Status."Close", "error in (no error)"=w466) -> ("VI out"=w468:refnum<vi>, "error out"=w469:errorcluster)  [unwired: 15 in]
            }
          }
          n170 = call "BaseProcess.set event status.vi"("i ref in"=w453, "EventStatus"=w458, "error in (no error)"=w454) -> ("i ref out"=w459:refnum<vi>, "error out"=w456:errorcluster)  [unwired: 14 in, 1 out]
          n171 = Unbundle By Name(w456) -> ("code"=w460:i32)
          n172 = case shown="No Error" w456 {
            selector: w456 -> [_ w473]
            tunnel: [T1 [] ("byteArray out") w471] -> w457
            frame No Error {
            }
            frame Error {
              n173 = Unbundle By Name(w473) -> ("source"=w472:string)
              n174 = call-poly "CoreLib.data 2 byte array.vi"("string"=w472) -> ("byteArray out"=w471:T1)  [unwired: 18 in]
            }
          }
          n175 = Bundle By Name(cluster=w462, "Data"=w457, "Error #"=w460) -> (w461:T2)
        }
        frame Default {
          n176 = call "PH_Stepmotor_BaseClass.ProcCases.vi"("i ref in"=w488, "selector"=w474, "Data"=w487, "call cluster"=w486, "error in"=w490) -> ("i ref out"=w475:refnum<vi>, "answer cluster"=w489:T2, "error out"=w480:errorcluster)  [unwired: 12 in]
          n177 = case shown="\"AbsoluteMove\", \"RelativeMove\"" w474 {
            tunnel: w480 -> [w491 w498]
            tunnel: [w491 w497] -> w477
            tunnel: [w492 w496] -> w476
            tunnel: w475 -> [w492 w494]
            frame Default {
            }
            frame "AbsoluteMove", "RelativeMove" {
              n178 = call "CSSystemLib.ref2name.vi"("obj refnum"=w494) -> ("name"=w493:string)
              n179 = call "BaseProcess.call process 2.vi"("i ref in"=w494, "Object"=w493, "Selector"="WakeupPeriodic", "error in (no error)"=w498) -> ("i ref out"=w496:refnum<vi>, "error out"=w497:errorcluster)  [unwired: 14 in]
            }
          }
          n180 = call "PH_Sixpack.handle Reset.vi"("VI in"=w476, "error in (no error)"=w477) -> ("VI out"=w478:refnum<vi>, "error out"=w479:errorcluster)  [unwired: 16 in]
          n181 = call "PH_Sixpack.Set BaseClass Changes to 6P Configuration.vi"("i ref in"=w478, "error in"=w479) -> ("i ref out"=w485:refnum<vi>, "Config changed?"=w481:bool, "error out"=w483:errorcluster)  [unwired: 15 in]
          n182 = call "PH_Sixpack.set Status Config changed.vi"("VI in"=w485, "Config changed?"=w481, "error in"=w483) -> ("VI out"=w484:refnum<vi>, "error out"=w482:errorcluster)  [unwired: 15 in]
        }
      }
    }
    frame Error {
    }
  }
  "answer cluster" <- w8
  "i ref out" <- w4
  "error out" <- w7
